vi "assembleVolume.vi"(6 "calc ff/fb":bool, 7 "tracking":bool, 8 "error in (no error)":errorcluster, 9 "xyz order":bool, 10 "Queues":T5) -> (0 "error out":errorcluster, 2 "sample volume to assemble":T1, 5 "status":T4)   [LabVIEW 2010]
uses:
  internal_queues.ctl
  line_info.ctl
  volume_with_lines.ctl
  volume_info.ctl
  kalman_result_scaled.ctl
  location3D.ctl
  spot location.ctl
  addLineToVolume.vi
  get write location linear fit.vi
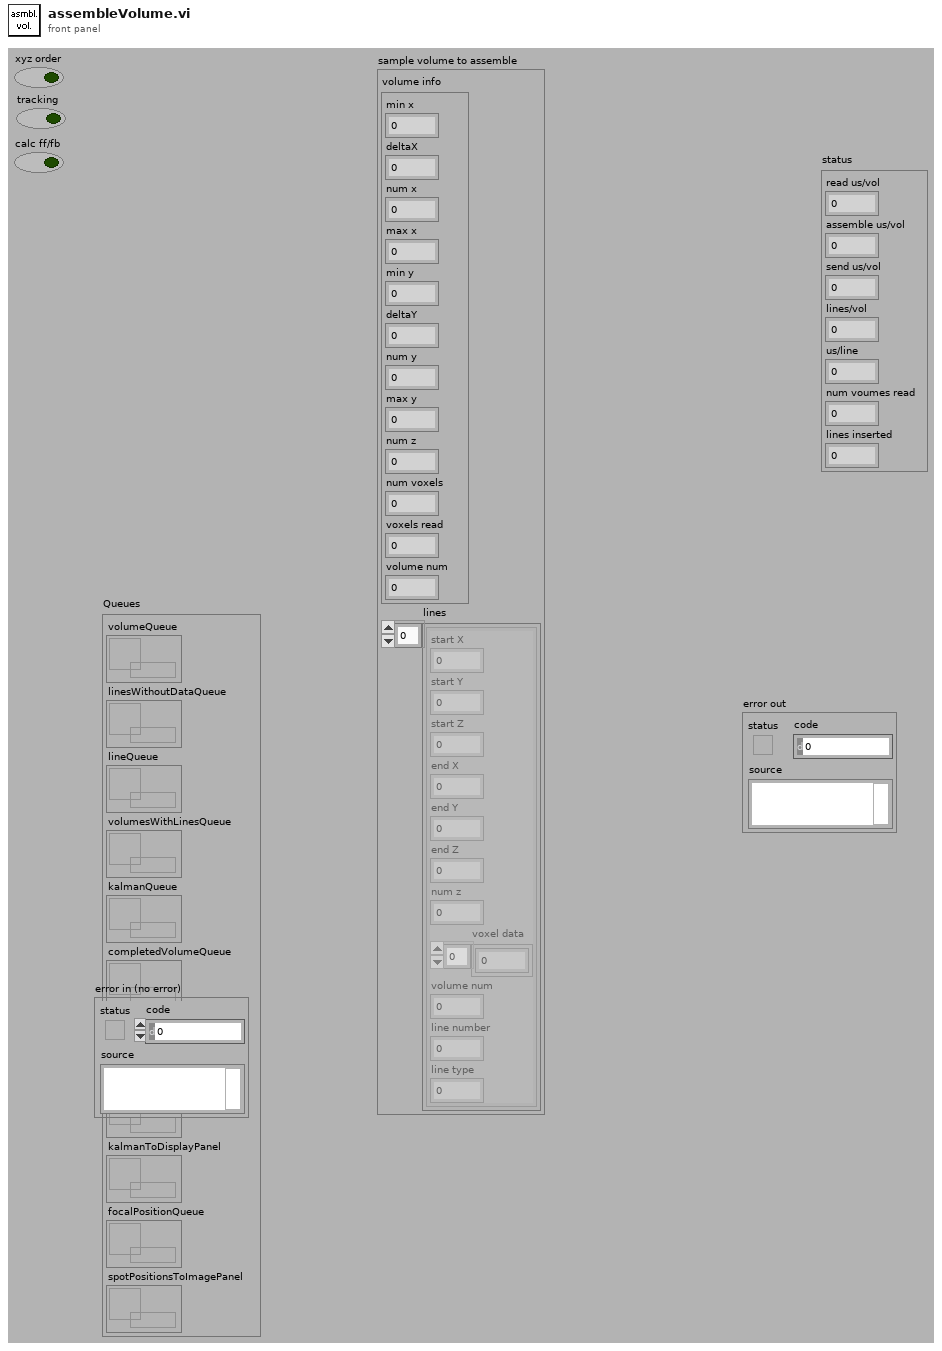
[diagram p1: front panel]
types:
  T1 = typedef "volume_with_lines.ctl" = cluster{"volume info":T2, "lines":T3[]}
  T2 = typedef "volume_info.ctl" = cluster{"min x":i16, "deltaX":dbl, "num x":u32, "max x":i16, "min y":i16, "deltaY":dbl, "num y":u32, "max y":i16, "num z":u32, "num voxels":u32, "voxels read":u32, "volume num":u32}
  T3 = typedef "line_info.ctl" = cluster{"start X":i16, "start Y":i16, "start Z":i16, "end X":i16, "end Y":i16, "end Z":i16, "num z":u8, "voxel data":u32[], "volume num":u32, "line number":u16, "line type":u16}
  T4 = cluster{"read us/vol":dbl, "assemble us/vol":dbl, "send us/vol":dbl, "lines/vol":dbl, "us/line":dbl, "num voumes read":u32, "lines inserted":i32}
  T5 = typedef "internal_queues.ctl" = cluster{"volumeQueue":refnum<queue>, "linesWithoutDataQueue":refnum<queue>, "lineQueue":refnum<queue>, "volumesWithLinesQueue":refnum<queue>, "kalmanQueue":refnum<queue>, "completedVolumeQueue":refnum<queue>, "displayVolumeQueue":refnum<queue>, "scanLocationsQueue":refnum<queue>, "kalmanToDisplayPanel":refnum<queue>, "focalPositionQueue":refnum<queue>, "spotPositionsToImagePanel":refnum<queue>}
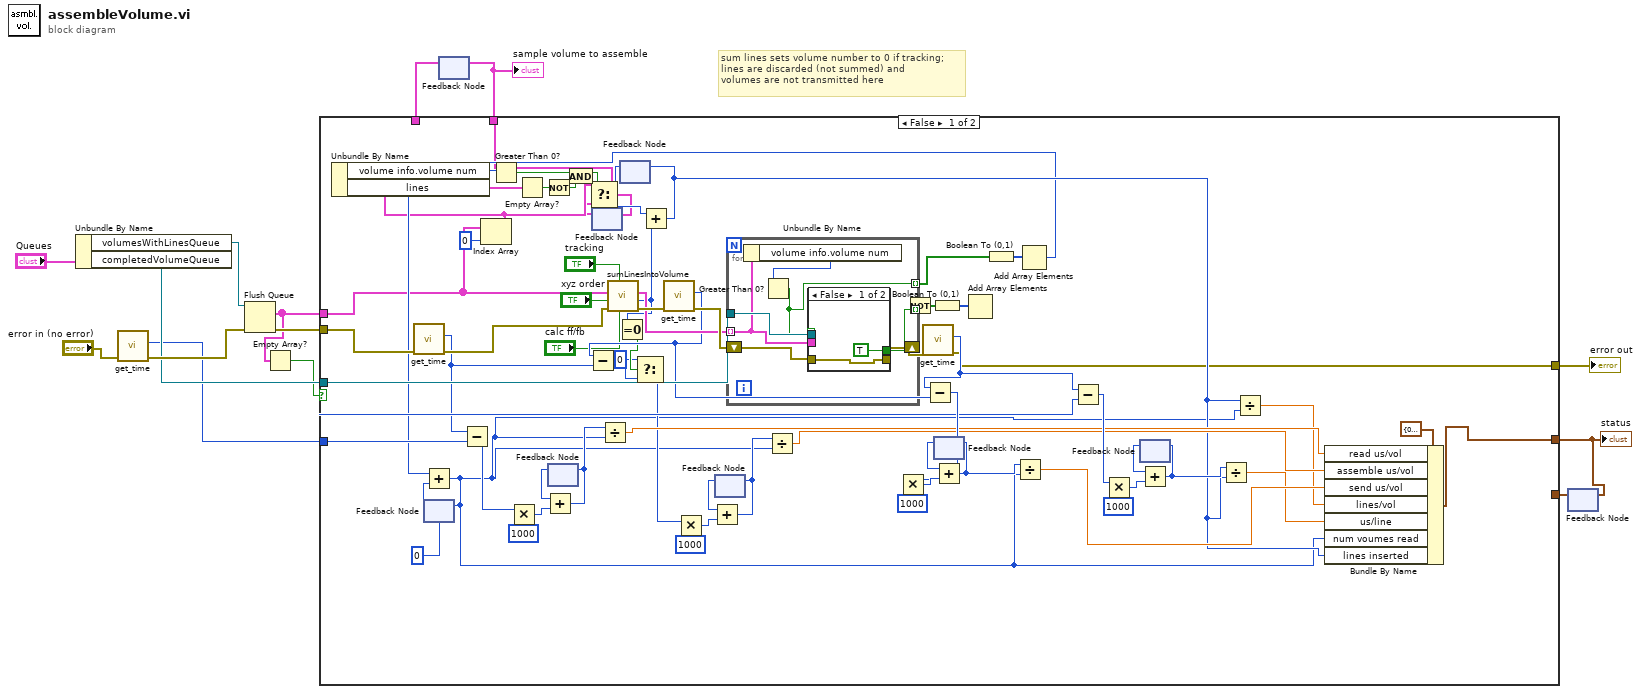
[diagram p0: block diagram]
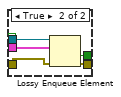
[diagram p2: hidden frame]
diagram:
  # "sum lines sets volume number to 0 if tracking;\nlines are discarded (not summed) and\nvolumes are not transmitted here"
  n1 = Unbundle By Name("Queues") -> ("volumesWithLinesQueue"=w14:refnum<queue>, "completedVolumeQueue"=w11:refnum<queue>)
  n2 = call "get_time.vi"("error in (no error)"="error in (no error)") -> ("error out"=w12:errorcluster, "millisecond timer value"=w10:u32)  [unwired: 9 in]
  n3 = Flush Queue(queue=w14, error in (no error)=w12) -> (remaining elements=w7:T1[], error out=w9:errorcluster)  [unwired: 1 out]
  n4 = Empty Array?(array=w7) -> (empty?=w6:bool)
  n5 = feedback #1() -> (w1:T1)  [unwired: 1 in]
  n6 = feedback #2() -> (w4:T4)  [unwired: 1 in]
  n7 = case shown="False" w6 {
    tunnel: w11 -> [w75 _]
    tunnel: w10 -> [w55 _]
    tunnel: w9 -> [w49 w98]
    tunnel: w7 -> [w25 _]
    tunnel: [w35 w99] -> w5
    tunnel: w4 -> [_ w99]
    tunnel: [w31 w98] -> w3
    tunnel: [w19 w97] -> w2
    tunnel: w1 -> [_ w97]
    frame False {
      n8 = call "get_time.vi"("error in (no error)"=w49) -> ("error out"=w48:errorcluster, "millisecond timer value"=w43:u32)  [unwired: 9 in]
      n9 = feedback #3(0) -> (w70:i32)
      n10 = Subtract(x=w43, y=w55) -> (x-y=w68:u32)
      n11 = Index Array(array=w25, index=0) -> (element=w21:T1)
      n12 = Unbundle By Name(w21) -> ("volume info.volume num"=w23:u32, "lines"=w18:T3[])
      n13 = Greater Than 0?(x=w23) -> (x > 0?=w22:bool)
      n14 = Multiply(x=w68, y=u32 1000 ("x")) -> (x*y=w81:u32)
      n15 = Empty Array?(array=w18) -> (empty?=w17:bool)
      n16 = Not(x=w17) -> (.not. x?=w15:bool)
      n17 = feedback #4() -> (w80:u32)  [unwired: 1 in]
      n18 = Add(x=w80, y=w81) -> (x+y=w79:u32)
      n19 = feedback-in #4(w79) -> ()
      n20 = And(x=w22, y=w15) -> (x .and. y?=w16:bool)
      n21 = feedback #5() -> (w20:T1)  [unwired: 1 in]
      n22 = Select(t=w21, s=w16, f=w20) -> (s? t:f=w19:T1)
      n23 = feedback-in #5(w19) -> ()
      n24 = call "sumLinesIntoVolume.vi"("calc ff/fb"="calc ff/fb", "tracking"="tracking", "error in (no error)"=w48, "xyz order"="xyz order", "volumes to assemble"=w25) -> ("error out"=w78:errorcluster, "lines inserted"=w40:i32, "volumes to send"=w76:cluster{"volume info":T2, u32[]}[])  [unwired: 4 in]
      n25 = Equal To 0?(x=w40) -> (x = 0?=w39:bool)
      n26 = feedback #6() -> (w47:i32)  [unwired: 1 in]
      n27 = Add(x=w47, y=w40) -> (x+y=w34:i32)
      n28 = feedback-in #6(w34) -> ()
      n29 = call "get_time.vi"("error in (no error)"=w78) -> ("error out"=w77:errorcluster, "millisecond timer value"=w58:u32)  [unwired: 9 in]
      n30 = Subtract(x=w58, y=w43) -> (x-y=w64:u32)
      n31 = Select(t=u32 0, s=w39, f=w64) -> (s? t:f=w41:u32)
      n32 = Multiply(x=w41, y=u32 1000 ("x")) -> (x*y=w66:u32)
      n33 = feedback #7() -> (w65:u32)  [unwired: 1 in]
      n34 = Add(x=w65, y=w66) -> (x+y=w63:u32)
      n35 = feedback-in #7(w63) -> ()
      n36 = for {
        tunnel: w76 -> [w85] mode=indexing
        tunnel: w75 -> [w89]
        shift-right: [w88] -> w71
        shift-left: w77 -> [w86]
        tunnel: [w87] -> w74 mode=indexing
        tunnel: [w83] -> w30 mode=indexing
        n37 = Unbundle By Name(w85) -> ("volume info.volume num"=w84:u32)
        n38 = Greater Than 0?(x=w84) -> (x > 0?=w83:bool)
        n39 = case shown="False" w83 {
          tunnel: w89 -> [_ w96]
          tunnel: [w90 w95] -> w88
          tunnel: [TRUE ("overflow?") w94] -> w87
          tunnel: w86 -> [w90 w93]
          tunnel: w85 -> [_ w92]
          frame False {
          }
          frame True {
            n40 = Lossy Enqueue Element(queue=w96, element=w92, error in (no error)=w93) -> (overflow?=w94:bool, error out=w95:errorcluster)  [unwired: 2 out]
          }
        }
      }
      n41 = Not(x=w74) -> (.not. x?=w73:bool[])
      n42 = call "get_time.vi"("error in (no error)"=w71) -> ("error out"=w31:errorcluster, "millisecond timer value"=w56:u32)  [unwired: 9 in]
      n43 = Subtract(x=w56, y=w58) -> (x-y=w57:u32)
      n44 = Multiply(x=w57, y=u32 1000 ("x")) -> (x*y=w62:u32)
      n45 = Boolean To (0,1)(Boolean=w73) -> (0, 1=w72:i16[])
      n46 = feedback #8() -> (w61:u32)  [unwired: 1 in]
      n47 = Add(x=w61, y=w62) -> (x+y=w59:u32)
      n48 = feedback-in #8(w59) -> ()
      n49 = Add Array Elements(numeric array=w72) -> ()  [unwired: 1 out]
      n50 = Boolean To (0,1)(Boolean=w30) -> (0, 1=w45:i16[])
      n51 = Add Array Elements(numeric array=w45) -> (sum=w33:i16)
      n52 = Add(x=w33, y=w70) -> (x+y=w29:i32)
      n53 = feedback-in #3(w29) -> ()
      n54 = Divide(x=w79, y=w29) -> (x/y=w44:dbl)
      n55 = Divide(x=w63, y=w29) -> (x/y=w42:dbl)
      n56 = Divide(x=w59, y=w29) -> (x/y=w37:dbl)
      n57 = Subtract(x=w56, y=w55) -> (x-y=w50:u32)
      n58 = Multiply(x=w50, y=u32 1000 ("x")) -> (x*y=w54:u32)
      n59 = feedback #9() -> (w53:u32)  [unwired: 1 in]
      n60 = Add(x=w53, y=w54) -> (x+y=w51:u32)
      n61 = feedback-in #9(w51) -> ()
      n62 = Divide(x=w51, y=w34) -> (x/y=w36:dbl)
      n63 = Divide(x=w34, y=w29) -> (x/y=w32:dbl)
      n64 = Bundle By Name(cluster=T4 {"read us/vol"=0.0, "assemble us/vol"=0.0, "send us/vol"=0.0, "lines/vol"=0.0, "us/line"=0.0, "num voumes read"=0, "lines inserted"=0} ("status"), "read us/vol"=w44, "assemble us/vol"=w42, "send us/vol"=w37, "lines/vol"=w32, "us/line"=w36, "num voumes read"=w29, "lines inserted"=w34) -> (w35:T4)
    }
    frame True {
    }
  }
  "status" <- w5
  "error out" <- w3
  "sample volume to assemble" <- w2
  n65 = feedback-in #1(w2) -> ()
  n66 = feedback-in #2(w5) -> ()
